vi "Actor Core.vi"(8 "error in":errorcluster, 11 "RP Delayed in":refnum<class "RP Level.lvclass">) -> (0 "error out":errorcluster, 3 "Actor out":refnum<class "Actor.lvclass">)   [LabVIEW 2018, in "RP Level.lvclass"]
doc: "(<B>Filename</B>: Actor Framework.lvlib:Actor.lvclass:Actor Core.vi)\n\nReceives messages to the actor, reacts to them, and initiates any error handling that may shut the actor down.\n\nDescendant classes may override this VI to append parallel tasks for the actor to complete while it handles messages. Overrides use the Call Parent Method node."
uses:
  RP Level.lvclass
  <vilib>/ActorFramework/Actor/Actor.lvclass
  NHMFL_Core/Libraries/Red Pitaya/RP Level Configuration.ctl
  Pulse Recorders/Pulse Recorder/Pulse Recorder.lvclass
panel:
  out "Armed":bool
  out "Name":string
  in  "Configuration":T1={"Pre-trigger duration"=0.01, "Post-trigger duration"=0.1, "Rate"=1000000.0, "Ranges"=[10.0], "Re-name channels"=[], "Active channels"="0:1", "External clock"=FALSE, "Output delay"=0.1, "Raising edge "=FALSE, "Trigger level"=0.001} {"Trigger level" format="%#_6pV"; "Output delay" format="%#_6ps"; "Rate" format="%#_8pHz"; "Post-trigger duration" format="%#_6ps"; "Pre-trigger duration" format="%#_6ps"; "Ranges" format="%#_6pV"}
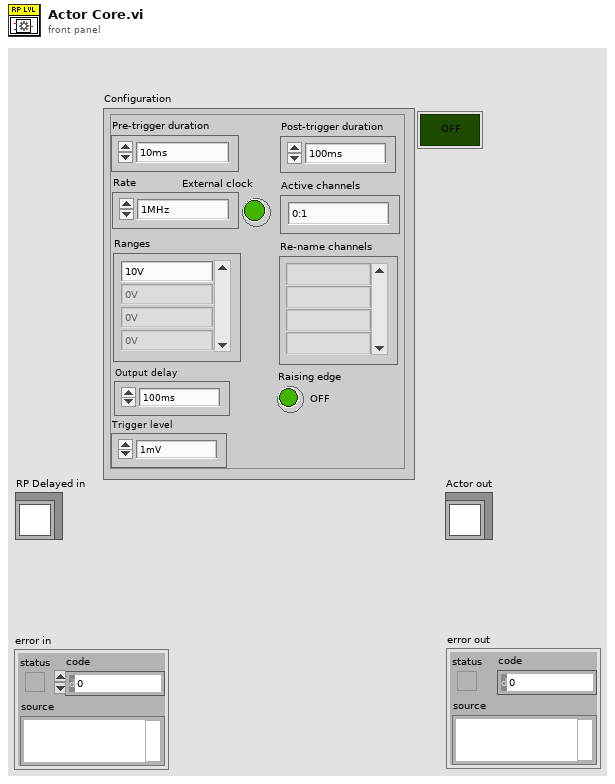
[diagram p1: front panel]
types:
  T1 = typedef "RP Level Configuration.ctl" = cluster{"Pre-trigger duration":dbl, "Post-trigger duration":dbl, "Rate":dbl, "Ranges":dbl[], "Re-name channels":string[], "Active channels":string, "External clock":bool, "Output delay":dbl, "Raising edge ":bool, "Trigger level":dbl}
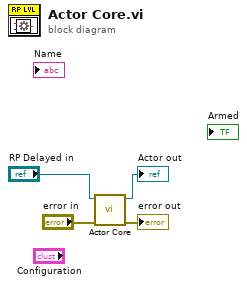
[diagram p0: block diagram]
diagram:
  n1 = call-parent "Actor Core.vi"("error in"="error in", "Pulse Recorder in"="RP Delayed in") -> ("error out"=→"error out":errorcluster, "Actor out"=→"Actor out":refnum<class "Actor.lvclass">)  [unwired: 8 in]
